vi "LV2 Object.vi"(0 "Add.lvclass":refnum<class "Add.lvclass">, 11 "Error in":errorcluster, 13 "Operations":T1) -> (4 "Add.lvclass":refnum<class "Add.lvclass">, 15 "Error out":errorcluster)   [LabVIEW 2020, in "Simple calculator.lvlib"]
uses:
  Simple calculator.lvlib
  Typedefs/Object LV2 operations.ctl
  Arithmetic Operations/Add/Add.lvclass
panel:
  # "Object LV2"
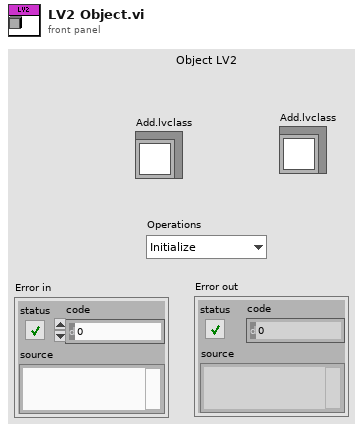
[diagram p1: front panel]
types:
  T1 = typedef "Simple calculator.lvlib/Object LV2 operations.ctl" = enum16{"Initialize", "Read", "Write"}
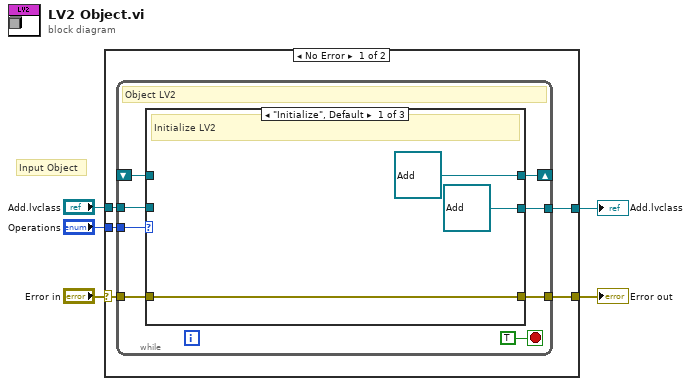
[diagram p0: block diagram]
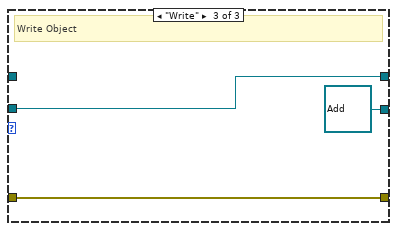
[diagram p3: hidden frame]
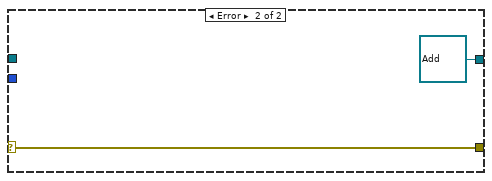
[diagram p4: hidden frame]
diagram:
  # "Input Object"
  n1 = case shown="No Error" "Error in" {
    selector: "Error in" -> [w10 w28]
    tunnel: [w9 w28] -> w4
    tunnel: "Operations" -> [w8 _]
    tunnel: "Add.lvclass" -> [w7 _]
    tunnel: [w6 refnum<class "Add.lvclass"> refnum ("Add.lvclass")] -> w1
    frame No Error {
      n2 = while {
        tunnel: w10 -> [w17]
        tunnel: [w16] -> w9
        tunnel: w8 -> [w15]
        shift-right: [w13] -> _
        shift-left: _ -> [w11]
        tunnel: w7 -> [w14]
        tunnel: [w12] -> w6
        stop <- TRUE stop-if-true
        # "Object LV2"
        n3 = case shown="\"Initialize\", Default" w15 {
          tunnel: [w21 w23 w26] -> w16
          tunnel: w17 -> [w21 w23 w26]
          tunnel: w14 -> [_ _ w25]
          tunnel: [refnum<class "Add.lvclass"> refnum ("Add.lvclass") w22 w25] -> w13
          tunnel: [refnum<class "Add.lvclass"> refnum ("Add.lvclass") w22 refnum<class "Add.lvclass"> refnum ("Add.lvclass")] -> w12
          tunnel: w11 -> [_ w22 _]
          frame "Initialize", Default {
            # "Initialize LV2"
          }
          frame "Read" {
            # "Read Object"
          }
          frame "Write" {
            # "Write Object"
          }
        }
      }
    }
    frame Error {
    }
  }
  "Error out" <- w4
  "Add.lvclass" <- w1
